vi "Log_Errors.vi"(7 "LoopName":string, 10 "error in":errorcluster) -> (2 "error out":errorcluster)   [LabVIEW 2018]
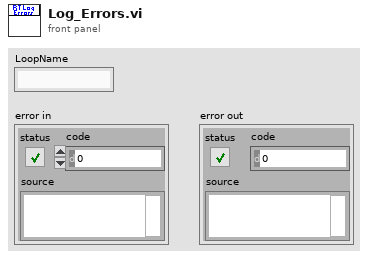
[diagram p1: front panel]
types:
  T1 = enum16{"open", "replace", "create", "open or create", "replace or create", "replace or create with confirmation"}
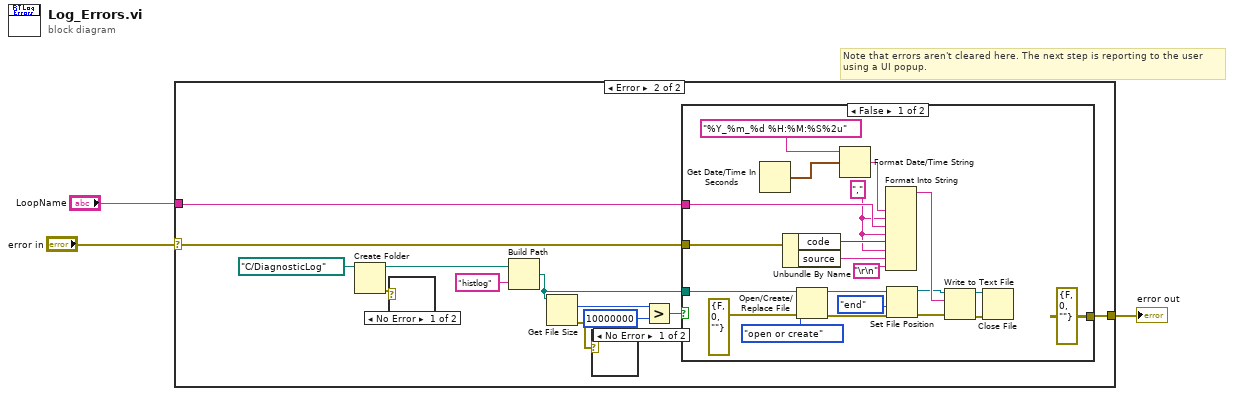
[diagram p0: block diagram]
diagram:
  # "Note that errors aren't cleared here. The next step is reporting to the user\nusing a UI popup."
  n1 = case shown="Error" "error in" {
    selector: "error in" -> [w4 w16]
    tunnel: [w4 w5] -> w2
    tunnel: "LoopName" -> [_ w15]
    frame No Error {
    }
    frame Error {
      n2 = Create Folder(path (use dialog)=path "C:/DiagnosticLog" ("file path (use dialog)")) -> (created path=w8:path, error out=w9:errorcluster)  [unwired: 2 in, 1 out]
      n3 = case shown="No Error" w9 {
        frame No Error {
        }
        frame Error {
        }
      }
      n4 = Build Path(base path=w8, name or relative path="histlog") -> (appended path=w6:path)
      n5 = Get File Size(file=w6) -> (size (in bytes)=w14:i64, 0:w11:errorcluster)  [unwired: 1 in, 1 out]
      n6 = case shown="No Error" w11 {
        frame No Error {
        }
        frame Error {
        }
      }
      n7 = Greater?(x=w14, y=i64 10000000) -> (0:w12:bool)
      n8 = case shown="False" w12 {
        tunnel: w16 -> [w18 w38]
        tunnel: w15 -> [w23 _]
        tunnel: w6 -> [w21 _]
        tunnel: [errorcluster {"status"=FALSE, "code"=0, "source"=""} ("error IO") w38] -> w5
        frame False {
          w22 = "," ("source")
          n9 = Get Date/Time In Seconds() -> (seconds since 1Jan1904=w36:timestamp)
          n10 = Unbundle By Name(w18) -> ("code"=w32:i32, "source"=w33:string)
          n11 = Open/Create/Replace File(file path (use dialog)=w21, error in=errorcluster {"status"=FALSE, "code"=0, "source"=""}, operation (0:open)=T1."open or create") -> (refnum out=w28:refnum<file>, error out=w25:errorcluster)  [unwired: 4 out]
          n12 = Format Date/Time String(time format string (%c)="%Y_%m_%d %H:%M:%S%2u", seconds (now)=w36) -> (date/time string=w37:string)  [unwired: 1 out]
          n13 = Format Into String(w37, w22, w23, w22, w32, w22, w33, "\r\n") -> (resulting string=w35:string)  [unwired: 3 in, 1 out]
          n14 = Set File Position(refnum=w28, from (0:start)=enum16{"start", "end", "current"}."end", error in=w25) -> (refnum out=w29:refnum<file>, error out=w26:errorcluster)  [unwired: 1 out]
          n15 = Write to Text File(file (use dialog)=w29, text=w35, error in=w26) -> (refnum out=w30:refnum<file>, error out=w27:errorcluster)  [unwired: 2 out]
          n16 = Close File(refnum=w30, error in=w27) -> ()  [unwired: 2 out]
        }
        frame True {
          # "Do not log errors if histlog file is greater than 500 kB.\nDo not let file grow unbounded.\nLuke 1/20/2014"
        }
      }
    }
  }
  "error out" <- w2
